vi "Launch Nested Panels.vi"(4 "Auto-stop? (T)":bool=TRUE, 6 "timeout in ms (-1)":i32=-1, 8 "error in (no error)":errorcluster, 10 "Nested Panel Actors":T1(array[cluster]), 11 "Panel Actor in":refnum<class "Panel Actor.lvclass">) -> (0 "error out":errorcluster, 1 "timed out?":bool, 2 "Nested Actor's Enqueuers":refnum<class "Message Enqueuer.lvclass">[](array[class]), 3 "Panel Actor out":refnum<class "Panel Actor.lvclass">)   [LabVIEW 2017, in "MGI-Panel Actor.lvlib" / "Panel Actor.lvclass"]
doc: "Launches multiple new nested Panle Actors with the specified Panel Type.\n\nThis method launches each panel serially, but waits for each one to be initialized in parallel.\n\n----\nCopyright: MGI 2018\nAuthor: Derek Trepanier"
uses:
  Panel Actor.lvclass
  <vilib>/ActorFramework/Actor/Actor.lvclass
  panel-manager/Source/Panel/Panel.lvclass
  panel-manager/Source/Init Waiter/Init Waiter.lvclass
  <vilib>/ActorFramework/Message Enqueuer/Message Enqueuer.lvclass
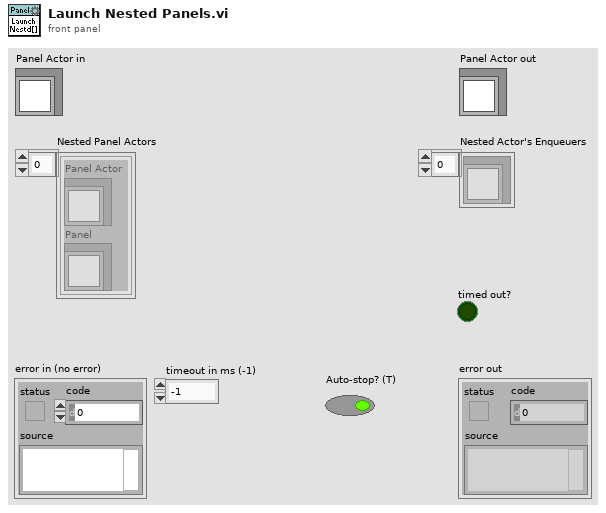
[diagram p1: front panel]
types:
  T1 = cluster{"Panel Actor":refnum<class "Panel Actor.lvclass">, "Panel":refnum<class "Panel.lvclass">}[]
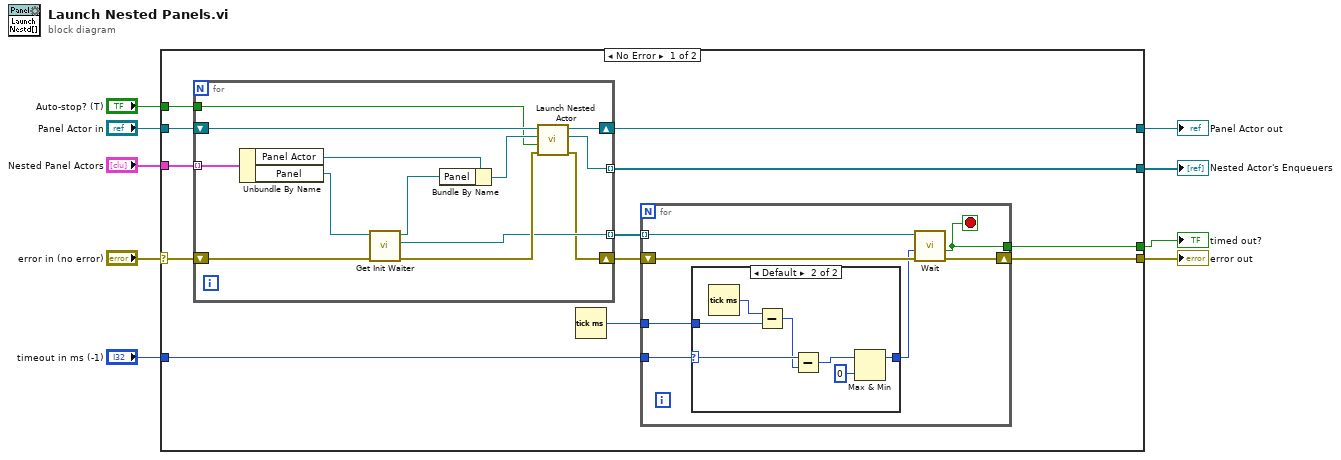
[diagram p0: block diagram]
diagram:
  n1 = case shown="No Error" "error in (no error)" {
    selector: "error in (no error)" -> [w16 w51]
    tunnel: [w14 w51] -> w8
    tunnel: [w19 w50] -> w6
    tunnel: "Panel Actor in" -> [w20 w50]
    tunnel: "Nested Panel Actors" -> [w21 _]
    tunnel: [w18 _] -> w1
    tunnel: "Auto-stop? (T)" -> [w17 _]
    tunnel: "timeout in ms (-1)" -> [w12 _]
    tunnel: [w11 _] -> w3
    frame No Error {
      n2 = for {
        tunnel: w21 -> [w49] mode=indexing
        tunnel: [w45] -> w18 mode=indexing
        tunnel: w17 -> [w44]
        tunnel: [w41] -> w15 mode=indexing
        shift-right: [w47] -> w19
        shift-left: w20 -> [w48]
        shift-right: [w40] -> w13
        shift-left: w16 -> [w43]
        n3 = Unbundle By Name(w49) -> ("Panel Actor"=w39:refnum<class "Panel Actor.lvclass">, "Panel"=w38:refnum<class "Panel.lvclass">)
        n4 = call "Get Init Waiter.vi"("Error In"=w43, "Panel In"=w38) -> ("Error Out"=w42:errorcluster, "Init Waiter"=w41:refnum<class "Init Waiter.lvclass">, "Panel Out"=w37:refnum<class "Panel.lvclass">)  [unwired: 7 in]
        n5 = Bundle By Name(cluster=w39, "Panel"=w37) -> (w46:refnum<class "Panel Actor.lvclass">)
        n6 = call <vilib>:"Launch Nested Actor.vi"("error in (no error)"=w42, "Auto-stop? (T)"=w44, "Nested Actor"=w46, "Caller Actor in"=w48) -> ("error out"=w40:errorcluster, "Nested Actor's Enqueuer"=w45:refnum<class "Message Enqueuer.lvclass">, "Caller Actor out"=w47:refnum<class "Panel Actor.lvclass">)  [unwired: 5 in]
      }
      n7 = Tick Count (ms)() -> (millisecond timer value=w10:u32)
      n8 = for {
        tunnel: w15 -> [w28] mode=indexing
        tunnel: w12 -> [w24]
        tunnel: [w22] -> w11
        shift-right: [w27] -> w14
        shift-left: w13 -> [w26]
        tunnel: w10 -> [w25]
        stop <- w22 stop-if-true
        n9 = case shown="Default" w24 {
          selector: w24 -> [w29 w34]
          tunnel: w25 -> [_ w35]
          tunnel: [w29 w32] -> w23
          frame -1 {
          }
          frame Default {
            n10 = Tick Count (ms)() -> (millisecond timer value=w36:u32)
            n11 = Subtract(x=w36, y=w35) -> (x-y=w33:i32)
            n12 = Subtract(x=w34, y=w33) -> (x-y=w31:i32)
            n13 = Max & Min(x=w31, y=0) -> (max(x,y)=w32:i32)  [unwired: 1 out]
          }
        }
        n14 = call "Wait.vi"("Error In"=w26, "timeout in ms (-1)"=w23, "Init Waiter in"=w28) -> ("Error Out"=w27:errorcluster, "timed out?"=w22:bool)  [unwired: 6 in, 1 out]
      }
    }
    frame Error {
    }
  }
  "error out" <- w8
  "Panel Actor out" <- w6
  "timed out?" <- w3
  "Nested Actor's Enqueuers" <- w1
